vi "ARydh_set_freq-and-get--V1.vi"(4 "Oscillator (0)":u16, 6 "delay-circle(msec)":i64, 8 "Error In":errorcluster, 9 "timeconstant (s)":dbl=0.006, 10 "Freq in (Hz)":dbl=40000.0 format="%#_13g", 11 "MCL object":T1) -> (0 "Error Out":errorcluster, 1 "z out (V)":cdb, 2 "Freq out (Hz)":dbl=40000.0 format="%#_13g", 3 "MCL object OUT":T1)   [LabVIEW 2020]
uses:
  <instrlib>/Zurich Instruments LabOne/Public/ziTypeHandle.ctl
  <instrlib>/Zurich Instruments LabOne/Zurich Instruments LabOne.lvlib
  nanocal/Nanocalorimetry/data/MCL.lvlibp/MCL library/MCL_DataRef.ctl
panel:
  out "Handle Out":T2 {"Handle" format="0x%08x"; "Conn" format="0x%08x"}
  in  "Handle In":T2 {"Handle" format="0x%08x"; "Conn" format="0x%08x"}
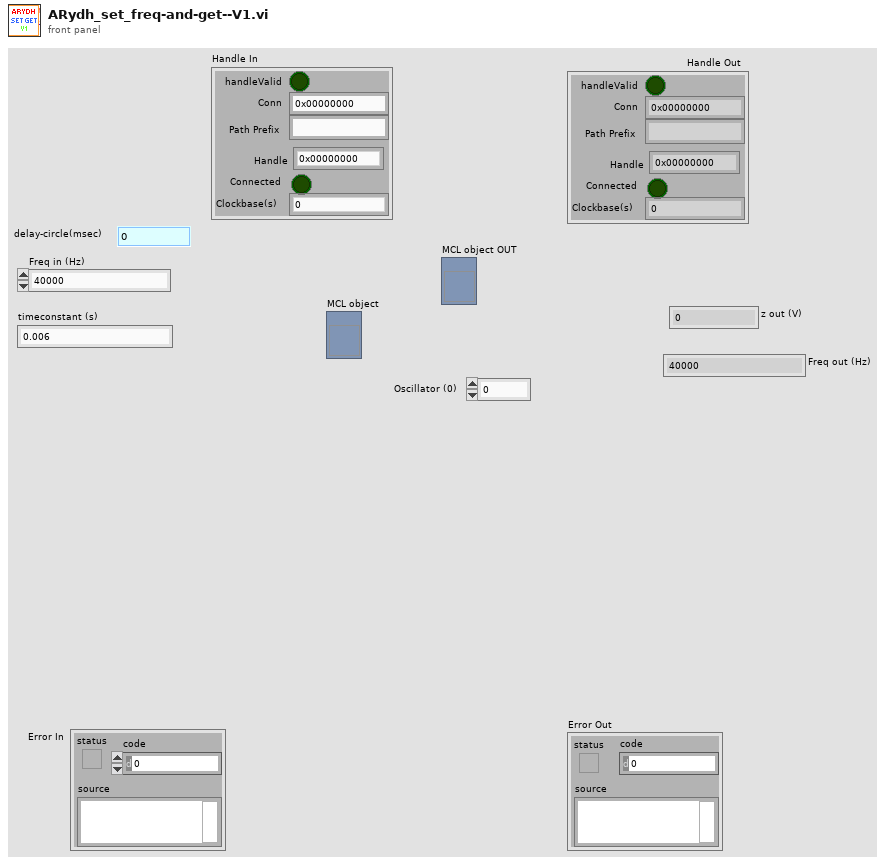
[diagram p1: front panel]
types:
  T1 = typedef "MCL.lvlibp/MCL_DataRef.ctl" = refnum<vi>
  T2 = typedef "Zurich Instruments LabOne.lvlib/ziTypeHandle.ctl" = cluster{"handleValid":bool, "Conn":u64, "Path Prefix":string, "Handle":u64, "Connected":bool, "Clockbase(s)":dbl}
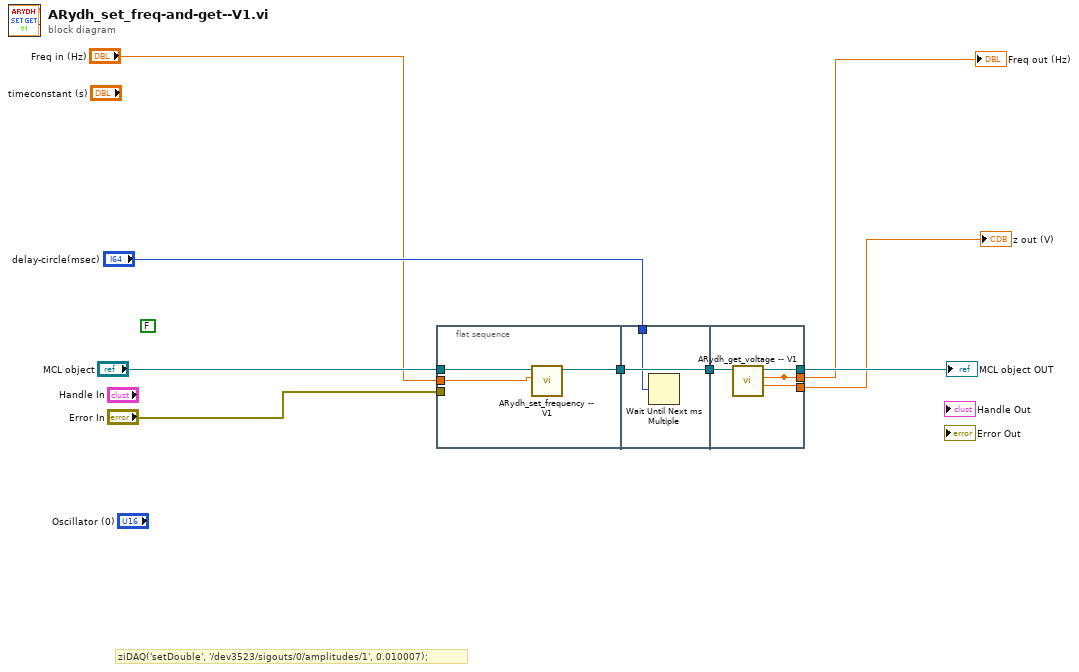
[diagram p0: block diagram]
diagram:
  (unwired) FALSE
  # "ziDAQ('setDouble', '/dev3523/sigouts/0/amplitudes/1', 0.010007);"
  n1 = flat-sequence {
    tunnel: "Freq in (Hz)" -> [w10]
    tunnel: "MCL object" -> [w11]
    tunnel: "Error In" -> [_]
    tunnel: [w12] -> w8
    tunnel: w8 -> [w14]
    tunnel: [w14] -> w7
    tunnel: "delay-circle(msec)" -> [w13]
    tunnel: [w17] -> w4
    tunnel: w7 -> [w18]
    tunnel: [w16] -> w2
    tunnel: [w15] -> _
    tunnel: [w15] -> w1
    frame #0 {
      n2 = call "ARydh_set_frequency -- V1.vi"("Freq in (Hz)"=w10, "MCL object"=w11) -> ("MCL object OUT"=w12:T1)  [unwired: 6 in, 3 out]
    }
    frame #1 {
      n3 = Wait Until Next ms Multiple(millisecond multiple=w13) -> ()  [unwired: 1 out]
    }
    frame #2 {
      n4 = call "ARydh_get_voltage -- V1.vi"("MCL object IN"=w18) -> ("z out (V)"=w16:cdb, "Freq out (Hz)"=w15:dbl, "MCL object OUT"=w17:T1)  [unwired: 7 in, 1 out]
    }
  }
  "z out (V)" <- w2
  "Freq out (Hz)" <- w1
  "MCL object OUT" <- w4
